vi "Error Code to Error Cluster.vi"(7 "Error Code":i32, 8 "Error Source":string, 13 "Error In":errorcluster) -> (2 "Error Out":errorcluster)   [LabVIEW 2021, in "Error.lvlib"]
uses:
  Error.lvlib
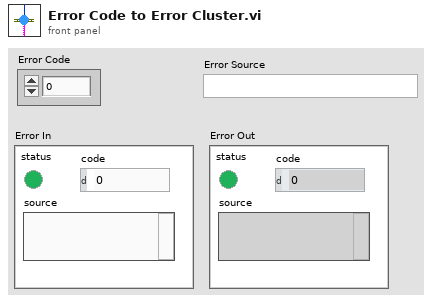
[diagram p1: front panel]
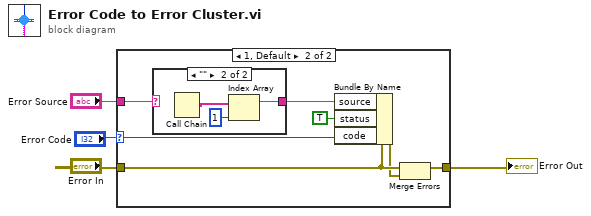
[diagram p0: block diagram]
diagram:
  n1 = case shown="1, Default" "Error Code" {
    selector: "Error Code" -> [_ w12]
    tunnel: "Error In" -> [w5 w8]
    tunnel: [w5 w9] -> w2
    tunnel: "Error Source" -> [_ w6]
    frame 0 {
    }
    frame 1, Default {
      n2 = case shown="\"\"" w6 {
        selector: w6 -> [w13 _]
        tunnel: [w13 w15] -> w10
        frame "not empty", Default {
        }
        frame "" {
          n3 = Call Chain() -> (call chain=w16:string[])
          n4 = Index Array(array=w16, index=1) -> (element=w15:string)
        }
      }
      n5 = Bundle By Name(cluster=w8, "source"=w10, "status"=TRUE, "code"=w12) -> (w7:errorcluster)
      n6 = Merge Errors(w8, w7) -> (w9:errorcluster)
    }
  }
  "Error Out" <- w2
